vi "Generated Data.vi"() -> ()   [LabVIEW 2014]
panel:
  out "Data":dbl
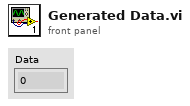
[diagram p1: front panel]
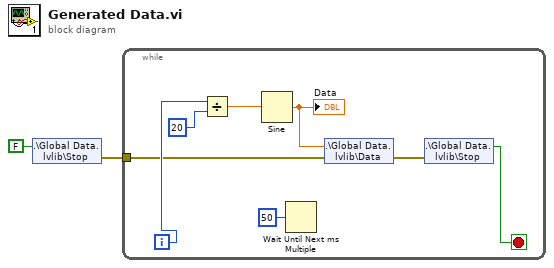
[diagram p0: block diagram]
diagram:
  n1 = shared-variable ".\\Global Data.lvlib\\Stop"(FALSE ("Stop")) -> (error out=w2:errorcluster)  [unwired: 1 in]
  n2 = while {
    tunnel: w2 -> [w3]
    i -> [w10]
    stop <- w5 stop-if-true
    n3 = Divide(x=w10, y=20) -> (x/y=w8:dbl)
    n4 = Sine(x=w8) -> (sin(x)=w6:dbl)
    "Data" <- w6
    n5 = Wait Until Next ms Multiple(millisecond multiple=u32 50) -> ()  [unwired: 1 out]
    n6 = shared-variable ".\\Global Data.lvlib\\Data"(w6, error in=w3) -> (error out=w4:errorcluster)
    n7 = shared-variable ".\\Global Data.lvlib\\Stop"(error in=w4) -> (w5:bool)  [unwired: 1 out]
  }
